vi "tcp_Example.vi"() -> ()   [LabVIEW 2020]
uses:
  controls/glbRoboterData.ctl
  <vilib>/Instr/_visa.llb/VISA Configure Serial Port (Instr).vi
panel:
  in  "Tab Control":enum32{"Page 1", "Page 2"}(tab)
  out "element":T1
  out "Chart":i16[][](graph)
  in  "VISA resource name":refnum<visa-resource-name>="COM5"
  out "Numeric":i32
  out "cycleTime (ms)":u32(graph)
  in  "milliseconds to wait":u32=50
  out "error out":errorcluster
  in  "stop":bool
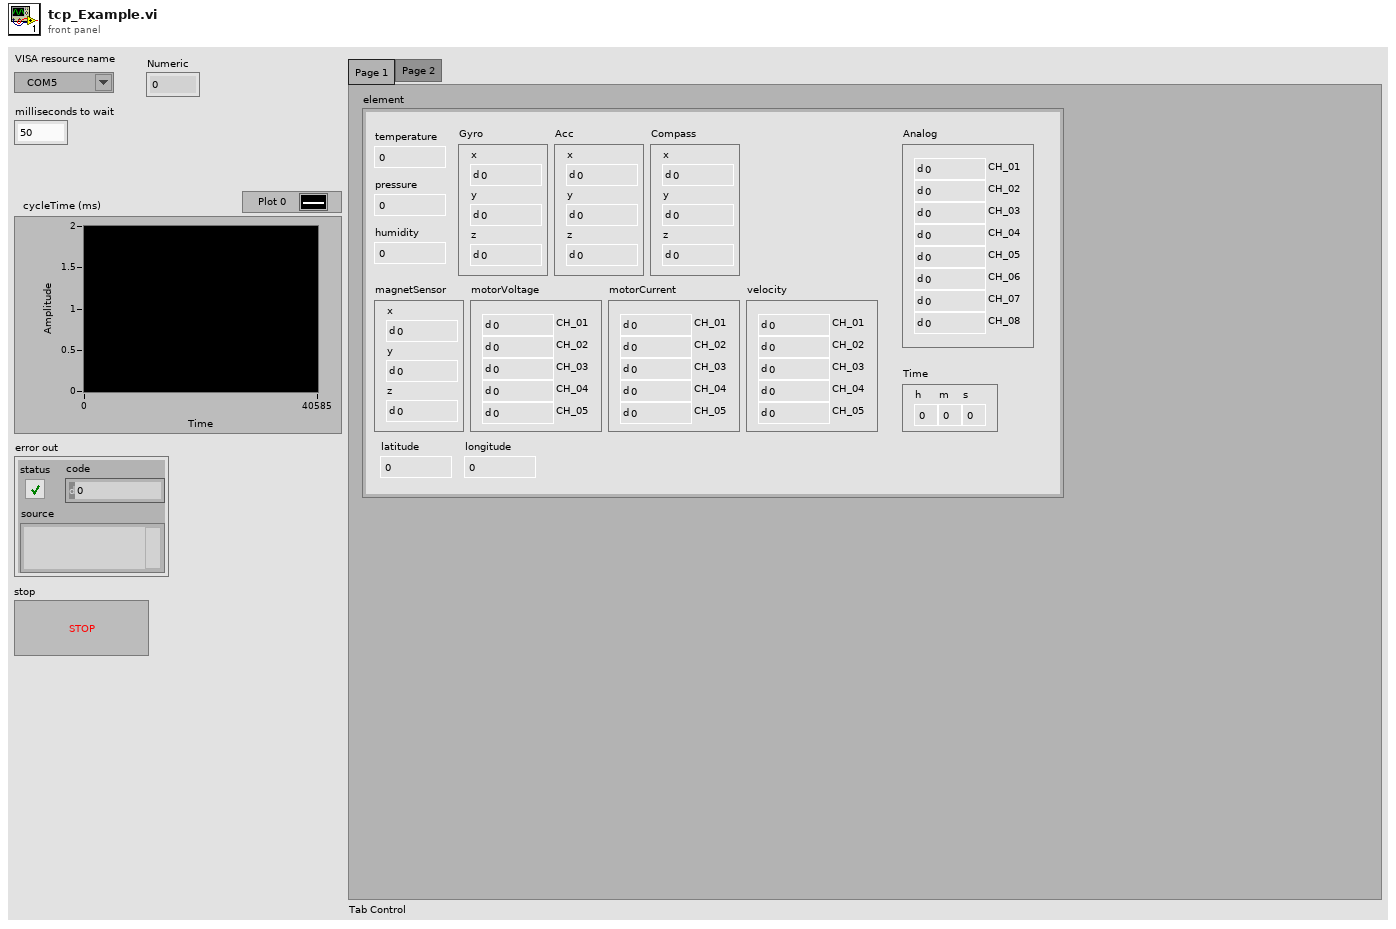
[diagram p1: front panel]
types:
  T1 = typedef "glbRoboterData.ctl" = cluster{"temperature":i16, "pressure":i16, "humidity":i16, "Gyro":cluster{"x":i16, "y":i16, "z":i16}, "Acc":cluster{"x":i16, "y":i16, "z":i16}, "Compass":cluster{"x":i16, "y":i16, "z":i16}, "Analog":cluster{"CH_01":i16, "CH_02":i16, "CH_03":i16, "CH_04":i16, "CH_05":i16, "CH_06":i16, "CH_07":i16, "CH_08":i16}, "magnetSensor":cluster{"x":i16, "y":i16, "z":i16}, "motorVoltage":cluster{"CH_01":i16, "CH_02":i16, "CH_03":i16, "CH_04":i16, "CH_05":i16}, "motorCurrent":cluster{"CH_01":i16, "CH_02":i16, "CH_03":i16, "CH_04":i16, "CH_05":i16}, "velocity":cluster{"CH_01":i16, "CH_02":i16, "CH_03":i16, "CH_04":i16, "CH_05":i16}, "latitude":sgl, "longitude":sgl, "Time":cluster{"h":u8, "m":u8, "s":u8}}
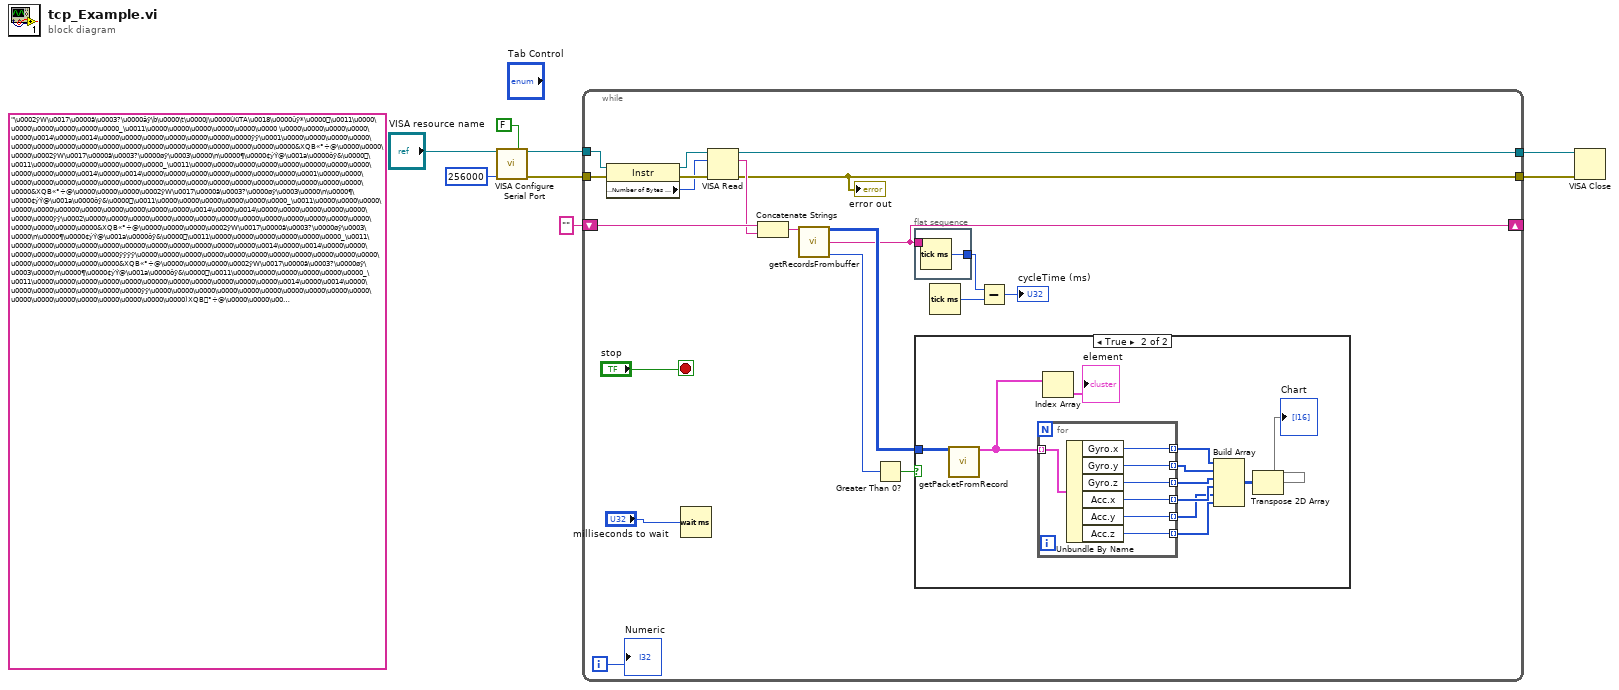
[diagram p0: block diagram]
diagram:
  (unwired) "\u0002ÿW\u0017\u0000ä\u0003?\u0000âÿ\b\u0000\t\u0000j\u0000ÙüTA\u0018\u0000ûÿ*\u0000\u0011\u0000\u0000\u0000\u0000\u0000\u0000_\u0011\u0000\u0000\u0000\u0000\u0000\u0000 \u0000\u0000\u0000\u0000\u0000\u0014\u0000\u0014\u0000\u0000\u0000\u0000\u0000\u0000\u0000ÿÿ\u0001\u0000\u0000\u0000\u0000\u0000\u0000\u0000\u0000\u0000\u0000\u0000\u0000\u0000\u0000\u0000\u0000\u0000&XQB«°÷@\u0000\u0000\u0000\u0002ÿW\u0017\u0000ä\u0003?\u0000øÿ\u0003\u0000\n\u0000¶\u0000¢ýÝ@\u001a\u0000ôÿ&\u0000\u0011\u0000\u0000\u0000\u0000\u0000\u0000_\u0011\u0000\u0000\u0000\u0000\u0000\u00000\u0000\u0000\u0000\u0000\u0000\u0014\u0000\u0014\u0000\u0000\u0000\u0000\u0000\u0000\u0000\u0001\u0000\u0000\u0000\u0000\u0000\u0000\u0000\u0000\u0000\u0000\u0000\u0000\u0000\u0000\u0000\u0000\u0000\u0000\u0000&XQB«°÷@\u0000\u0000\u0000\u0002ÿW\u0017\u0000ä\u0003?\u0000øÿ\u0003\u0000\n\u0000¶\u0000¢ýÝ@\u001a\u0000ôÿ&\u0000\u0011\u0000\u0000\u0000\u0000\u0000\u0000_\u0011\u0000\u0000\u0000\u0000\u0000\u00000\u0000\u0000\u0000\u0000\u0000\u0014\u0000\u0014\u0000\u0000\u0000\u0000\u0000\u0000\u0000ÿÿ\u0002\u0000\u0000\u0000\u0000\u0000\u0000\u0000\u0000\u0000\u0000\u0000\u0000\u0000\u0000\u0000\u0000\u0000&XQB«°÷@\u0000\u0000\u0000\u0002ÿW\u0017\u0000ä\u0003?\u0000øÿ\u0003\u0000\n\u0000¶\u0000¢ýÝ@\u001a\u0000ôÿ&\u0000\u0011\u0000\u0000\u0000\u0000\u0000\u0000_\u0011\u0000\u0000\u0000\u0000\u0000\u00000\u0000\u0000\u0000\u0000\u0000\u0014\u0000\u0014\u0000\u0000\u0000\u0000\u0000\u0000\u0000ÿÿÿÿ\u0000\u0000\u0000\u0000\u0000\u0000\u0000\u0000\u0000\u0000\u0000\u0000\u0000\u0000\u0000\u0000&XQB«°÷@\u0000\u0000\u0000\u0002ÿW\u0017\u0000ä\u0003?\u0000øÿ\u0003\u0000\n\u0000¶\u0000¢ýÝ@\u001a\u0000ôÿ&\u0000\u0011\u0000\u0000\u0000\u0000\u0000\u0000_\u0011\u0000\u0000\u0000\u0000\u0000\u00000\u0000\u0000\u0000\u0000\u0000\u0014\u0000\u0014\u0000\u0000\u0000\u0000\u0000\u0000\u0000ÿÿ\u0000\u0000\u0000\u0000\u0000\u0000\u0000\u0000\u0000\u0000\u0000\u0000\u0000\u0000\u0000\u0000\u0000\u0000)XQB°÷@\u0000\u0000\u0000\u0002ÿW\u0017\u0000ä\u0003?\u0000úÿ\u0005\u0000\u0007\u0000Ö\u0000Ùý¶@\u0017\u0000õÿ+\u0000\u0011\u0000\u0000\u0000\u0000\u0000\u0000^\u0011\u0000\u0000\u0000\u0000\u0000\u0000p\u0000\u0000\u0000\u0000\u0000\u0014\u0000\u0014\u0000\u0000\u0000\u0000\u0000\u0000\u0000\u0002\u0000\u0001\u0000\u0000\u0000\u0000\u0000\u0000\u0000\u0000\u0000\u0000\u0000\u0000\u0000\u0000\u0000\u0000\u0000)XQB°÷@\u0000\u0000\u0000\u0002ÿW\u0017\u0000ä\u0003?\u0000úÿ\u0005\u0000\u0007\u0000Ö\u0000Ùý¶@\u0017\u0000õÿ+\u0000\u0011\u0000\u0000\u0000\u0000\u0000\u0000^\u0011\u0000\u0000\u0000\u0000\u0000\u0000p\u0000\u0000\u0000\u0000\u0000\u0014\u0000\u0014\u0000\u0000\u0000\u0000\u0000\u0000\u0000\u0001..." ("concatenated string")
  n1 = call-poly "VISA Configure Serial Port"("VISA resource name"="VISA resource name", "Enable Termination\nChar (T)"=FALSE ("Enable Termination\nChar (T)"), "baud rate (9600)"=u32 256000) -> ("VISA resource name out"=w7:refnum<visa-resource-name>, "error out"=w6:errorcluster)  [unwired: 11 in]
  n2 = while {
    shift-right: [w23] -> _
    shift-left: "" ("remaining data") -> [w21]
    tunnel: w7 -> [w19]
    tunnel: w6 -> [w20]
    tunnel: [w13] -> w2
    tunnel: [w12] -> w1
    i -> [w22]
    stop <- "stop" stop-if-true
    n3 = property class="Instr"(reference=w19, error in=w20) -> (reference out=w18:refnum<visa-resource-name>, error out=w17:errorcluster, "Serial Settings:Number of Bytes at Serial Port"=w16:u32)
    n4 = Wait (ms)(milliseconds to wait="milliseconds to wait") -> ()  [unwired: 1 out]
    n5 = VISA Read(VISA resource name=w18, byte count=w16, error in (no error)=w17) -> (VISA resource name out=w13:refnum<visa-resource-name>, read buffer=w14:string, error out=w12:errorcluster)  [unwired: 1 out]
    "error out" <- w12
    n6 = Concatenate Strings(w21, w14) -> (w15:string)
    n7 = call "getRecordsFrombuffer.vi"("data in"=w15) -> ("foundPack"=w24:u8[][], "remaining data"=w23:string, "Found"=w10:i32)  [unwired: 10 in, 2 out]
    n8 = Greater Than 0?(x=w10) -> (x > 0?=w9:bool)
    n9 = flat-sequence {
      tunnel: [w47] -> w27
      tunnel: w23 -> [_]
      frame #0 {
        n10 = Tick Count (ms)() -> (millisecond timer value=w47:u32)
      }
    }
    n11 = case shown="True" w9 {
      tunnel: w24 -> [_ w39]
      frame False {
      }
      frame True {
        n12 = call "getPacketFromRecord.vi"("foundPack"=w39) -> ("PacketArray"=w38:T1[])  [unwired: 14 in]
        n13 = for {
          tunnel: w38 -> [w46] mode=indexing
          tunnel: [w45] -> w36 mode=indexing
          tunnel: [w44] -> w35 mode=indexing
          tunnel: [w43] -> w34 mode=indexing
          tunnel: [w42] -> w33 mode=indexing
          tunnel: [w41] -> w32 mode=indexing
          tunnel: [w40] -> w31 mode=indexing
          n14 = Unbundle By Name(w46) -> ("Gyro.x"=w45:i16, "Gyro.y"=w44:i16, "Gyro.z"=w43:i16, "Acc.x"=w42:i16, "Acc.y"=w41:i16, "Acc.z"=w40:i16)
        }
        n15 = Index Array(array=w38) -> (element=→"element":T1)  [unwired: 1 in]
        n16 = Build Array(w36, w35, w34, w33, w32, w31) -> (w30:i16[][])
        n17 = Transpose 2D Array(2D array=w30) -> (transposed array=→"Chart":i16[][])
      }
    }
    n18 = Tick Count (ms)() -> (millisecond timer value=w28:u32)
    n19 = Subtract(x=w27, y=w28) -> (x-y=→"cycleTime (ms)":u32)
    "Numeric" <- w22
  }
  n20 = VISA Close(VISA resource name=w2, error in (no error)=w1) -> ()  [unwired: 1 out]
